vi "WM Wave Height to Stroke.vi"(1 "Water Depth (m)":dbl format="%.2f", 2 "Flap Height (m)":dbl=3.3147 format="%.4f", 3 "Wave Period (s)":dbl format="%.2f", 4 "Wave Height (m)":dbl format="%.2f") -> (0 "Flap Amplitude (from x=0) (m)":dbl format="%.2f")   [LabVIEW 2012]
panel:
  # "Flap Stroke at Water line (S)"
  # "Flap Amplitude From x=0 (A')"
  # "Total Flap Stroke (S')"
  # "Flap Height (h')"
  # "Wave Height (Peak to trough) (H)"
  # "Wave Amplitude (z=0 to Peak) (A)"
  # "Wave Height to Flap Stroke at Water Line ( [H/S] )"
  # "Water Depth (h)"
  # "A' = h' * H / ( 2 * h * [H/S] )"
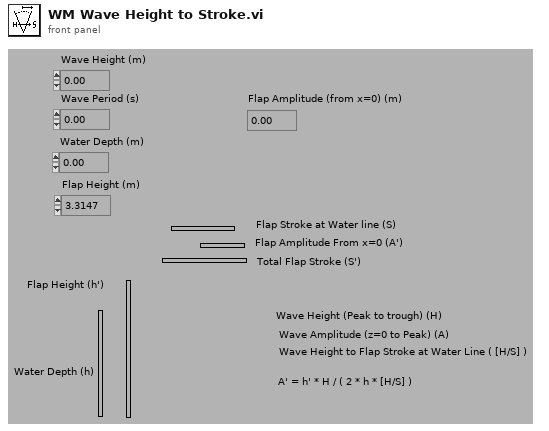
[diagram p1: front panel]
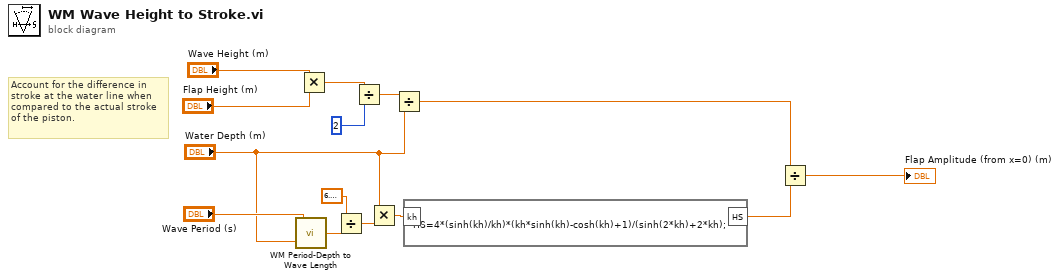
[diagram p0: block diagram]
diagram:
  # "Account for the difference in \nstroke at the water line when \ncompared to the actual stroke\nof the piston."
  n1 = call "WM Period-Depth to Wave Length.vi"("Water Depth"="Water Depth (m)", "Period"="Wave Period (s)") -> ("WaveLength"=w13:dbl)
  n2 = Multiply(x="Wave Height (m)", y="Flap Height (m)") -> (x*y=w8:dbl)
  n3 = Divide(x=6.283185307179586, y=w13) -> (x/y=w12:dbl)
  n4 = Divide(x=w8, y=2) -> (x/y=w5:dbl)
  n5 = Multiply(x="Water Depth (m)", y=w12) -> (x*y=w11:dbl)
  n6 = Divide(x=w5, y="Water Depth (m)") -> (x/y=w3:dbl)
  n7 = formula code="HS=4*(sinh(kh)/kh)*(kh*sinh(kh)-cosh(kh)+1)/(sinh(2*kh)+2*kh);"("kh"=w11) -> ("HS"=w4:dbl)
  n8 = Divide(x=w3, y=w4) -> (x/y=→"Flap Amplitude (from x=0) (m)":dbl)
